vi "CheckNextSnakeTile.vi"(9 "Direction (old)":T2, 10 "new position in":cluster{"row":i32, "col":i32}, 11 "Board in":T1[][](array[typedef])) -> (1 "Stop":bool, 2 "Tile":T1, 3 "Board out":T1[][](array[typedef]))   [LabVIEW 2020]
uses:
  TypeDef/direction.ctl
  TypeDef/tiles-key-trunct.ctl
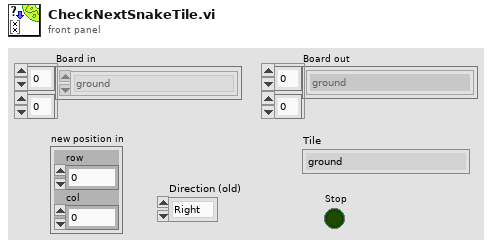
[diagram p1: front panel]
types:
  T1 = typedef "tiles-key-trunct.ctl" = enum16{"ground", "wall", "head (right)", "head (up)", "head (left)", "head (down)", "L-turn (right-up)", "L-turn (up-left)", "L-turn (left-down)", "L-turn (down-right)", "body (right)", "body (up)", "body (left)", "body (down)", "R-turn (right-down)", "R-turn (up-right)", "R-turn (left-up)", "R-turn (down-left)", "tail (right)", "tail (up)", "tail (left)", "tail (down)"}
  T2 = typedef "direction.ctl" = enum16{"Right", "Up", "Left", "Down"}
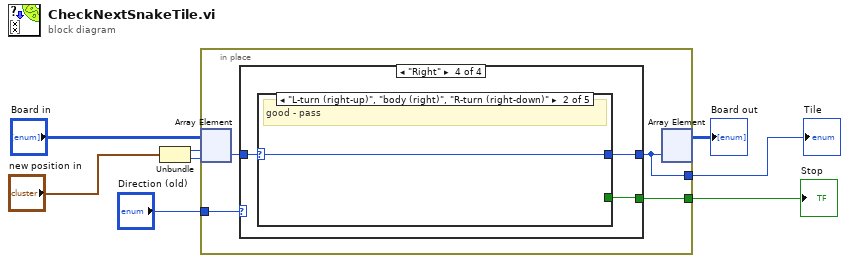
[diagram p0: block diagram]
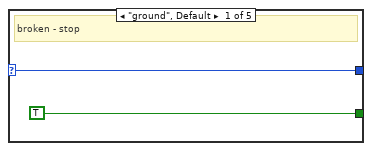
[diagram p3: hidden frame]
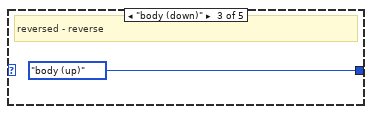
[diagram p4: hidden frame]
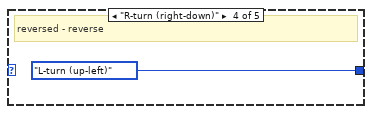
[diagram p5: hidden frame]
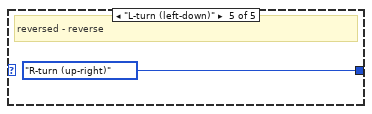
[diagram p6: hidden frame]
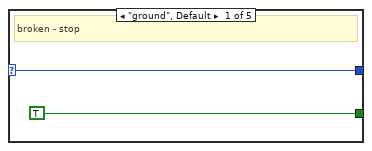
[diagram p8: hidden frame]
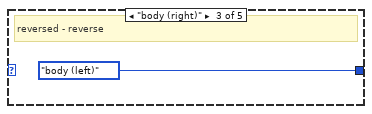
[diagram p9: hidden frame]
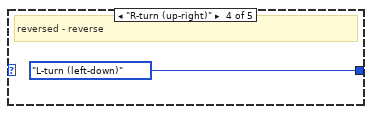
[diagram p10: hidden frame]
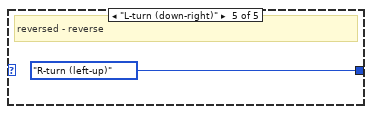
[diagram p11: hidden frame]
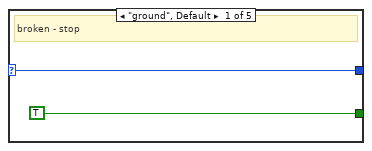
[diagram p13: hidden frame]
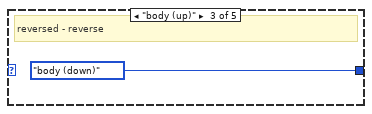
[diagram p14: hidden frame]
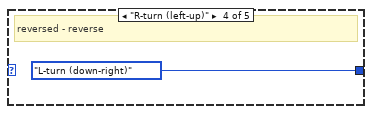
[diagram p15: hidden frame]
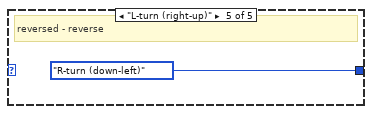
[diagram p16: hidden frame]
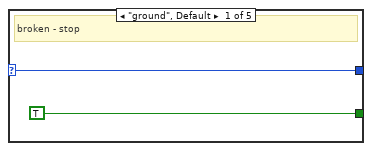
[diagram p17: hidden frame]
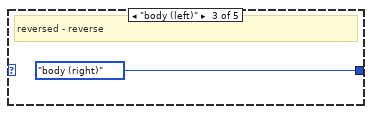
[diagram p18: hidden frame]
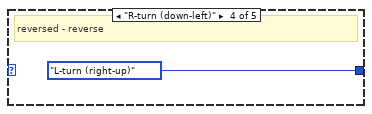
[diagram p19: hidden frame]
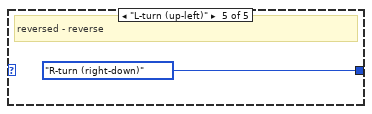
[diagram p20: hidden frame]
diagram:
  n1 = Unbundle("new position in") -> ("row"=w5:i32, "col"=w4:i32)
  n2 = in-place {
    in-place-border: "Direction (old)" -> [w12]
    in-place-border: [w10] -> w3
    in-place-border: [w9] -> w2
    n3 = in-place-array #1("Board in", w5, w4) -> (w11:T1)
    n4 = case shown="\"Right\"" w12 {
      tunnel: [w15 w24 w33 w42] -> w9
      tunnel: [w14 w23 w32 w41] -> w10
      tunnel: w11 -> [w13 w22 w31 w40]
      frame "Up" {
        n5 = case shown="\"L-turn (up-left)\", \"body (up)\", \"R-turn (up-right)\"" w13 {
          selector: w13 -> [w17 w18 _ _ _]
          tunnel: [w17 w18 tiles-key-trunct."body (up)" ("Tiles-key") tiles-key-trunct."L-turn (up-left)" ("Tiles-key") tiles-key-trunct."R-turn (up-right)" ("Tiles-key")] -> w15
          tunnel: [TRUE _ _ _ _] -> w14
          frame "ground", Default {
            # "broken - stop"
          }
          frame "L-turn (up-left)", "body (up)", "R-turn (up-right)" {
            # "good - pass"
          }
          frame "body (down)" {
            # "reversed - reverse"
          }
          frame "R-turn (right-down)" {
            # "reversed - reverse"
          }
          frame "L-turn (left-down)" {
            # "reversed - reverse"
          }
        }
      }
      frame "Left" {
        n6 = case shown="\"L-turn (left-down)\", \"body (left)\", \"R-turn (left-up)\"" w22 {
          selector: w22 -> [w26 w27 _ _ _]
          tunnel: [w26 w27 tiles-key-trunct."body (left)" ("Tiles-key") tiles-key-trunct."L-turn (left-down)" ("Tiles-key") tiles-key-trunct."R-turn (left-up)" ("Tiles-key")] -> w24
          tunnel: [TRUE _ _ _ _] -> w23
          frame "ground", Default {
            # "broken - stop"
          }
          frame "L-turn (left-down)", "body (left)", "R-turn (left-up)" {
            # "good - pass"
          }
          frame "body (right)" {
            # "reversed - reverse"
          }
          frame "R-turn (up-right)" {
            # "reversed - reverse"
          }
          frame "L-turn (down-right)" {
            # "reversed - reverse"
          }
        }
      }
      frame "Down" {
        n7 = case shown="\"L-turn (down-right)\", \"body (down)\", \"R-turn (down-left)\"" w31 {
          selector: w31 -> [w35 w36 _ _ _]
          tunnel: [w35 w36 tiles-key-trunct."body (down)" ("Tiles-key") tiles-key-trunct."L-turn (down-right)" ("Tiles-key") tiles-key-trunct."R-turn (down-left)" ("Tiles-key")] -> w33
          tunnel: [TRUE _ _ _ _] -> w32
          frame "ground", Default {
            # "broken - stop"
          }
          frame "L-turn (down-right)", "body (down)", "R-turn (down-left)" {
            # "good - pass"
          }
          frame "body (up)" {
            # "reversed - reverse"
          }
          frame "R-turn (left-up)" {
            # "reversed - reverse"
          }
          frame "L-turn (right-up)" {
            # "reversed - reverse"
          }
        }
      }
      frame "Right" {
        n8 = case shown="\"L-turn (right-up)\", \"body (right)\", \"R-turn (right-down)\"" w40 {
          selector: w40 -> [w44 w45 _ _ _]
          tunnel: [w44 w45 tiles-key-trunct."body (right)" ("Tiles-key") tiles-key-trunct."L-turn (right-up)" ("Tiles-key") tiles-key-trunct."R-turn (right-down)" ("Tiles-key")] -> w42
          tunnel: [TRUE _ _ _ _] -> w41
          frame "ground", Default {
            # "broken - stop"
          }
          frame "L-turn (right-up)", "body (right)", "R-turn (right-down)" {
            # "good - pass"
          }
          frame "body (left)" {
            # "reversed - reverse"
          }
          frame "R-turn (down-left)" {
            # "reversed - reverse"
          }
          frame "L-turn (up-left)" {
            # "reversed - reverse"
          }
        }
      }
    }
    n9 = in-place-array #1(w9) -> (→"Board out":T1[][])  [unwired: 2 out]
  }
  "Stop" <- w3
  "Tile" <- w2
